vi "Handle.vi"(7 "Event in":refnum<class "Event.lvclass">, 11 "State in":refnum<class "State.lvclass">) -> (2 "Destroy?":bool, 5 "Event out":refnum<class "Event.lvclass">)   [LabVIEW 2021, in "jettl.lvlib" / "Base Event.lvlib" / "State.lvlib" / "State.lvclass"]
uses:
  State.lvclass
  Event/Event.lvclass
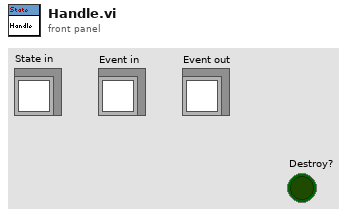
[diagram p1: front panel]
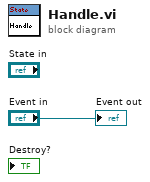
[diagram p0: block diagram]
diagram:
  "Event out" <- "Event in"
